vi "StartTrial.vi"(8 "error in (no error)":errorcluster, 11 "TrialBasedExperiment in":refnum<class "WNOriDiscExperiment.lvclass">) -> (0 "error out":errorcluster, 3 "TrialBasedExperiment out":refnum<class "WNOriDiscExperiment.lvclass">)   [LabVIEW 2014, in "WNOriDiscExperiment.lvclass"]
uses:
  WNOriDiscExperiment.lvclass
  WNOriDiscExperiment.lvclass/WNOriDiscExperiment.ctl
  TwoAfcEye/TwoAfcEye.lvclass
panel:
  in  "punishTime":dbl
  in  "cueTime":dbl
  in  "correctTargetOnly":bool
  in  "classOverride":bool
  in  "classShown":bool
  in  "punishType":string(combo)="None"
  in  "condRepeatType":string(combo)="None"
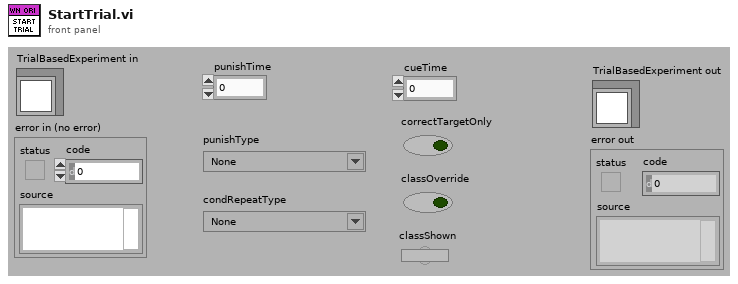
[diagram p1: front panel]
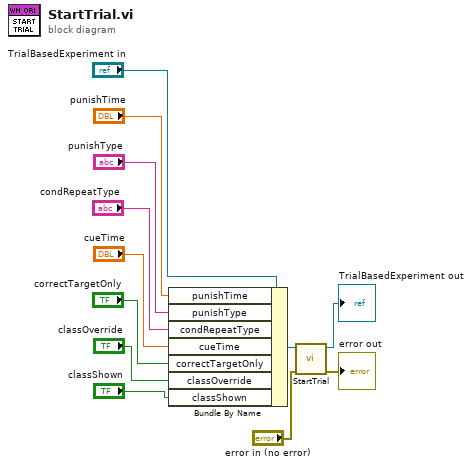
[diagram p0: block diagram]
diagram:
  n1 = Bundle By Name(cluster="TrialBasedExperiment in", "punishTime"="punishTime", "punishType"="punishType", "condRepeatType"="condRepeatType", "cueTime"="cueTime", "correctTargetOnly"="correctTargetOnly", "classOverride"="classOverride", "classShown"="classShown") -> (w10:refnum<class "WNOriDiscExperiment.lvclass">)
  n2 = call-parent "StartTrial.vi"("error in (no error)"="error in (no error)", "TrialBasedExperiment in"=w10) -> ("error out"=→"error out":errorcluster, "TrialBasedExperiment out"=→"TrialBasedExperiment out":refnum<class "WNOriDiscExperiment.lvclass">)  [unwired: 8 in]
